vi "Configure Volume.vi"(7 "Save":bool, 8 "error in (no error)":errorcluster, 9 "NumReps":i32, 10 "Scan Settings":T1, 11 "AODAcq in":refnum<class "AODAcq.lvclass">) -> (0 "error out":errorcluster, 3 "AODAcq out":refnum<class "AODAcq.lvclass">)   [LabVIEW 2011, in "AODAcq.lvclass"]
uses:
  AODAcq.lvclass
  <vilib>/rvi/interface/nirviReadWriteControl/nirviReadWriteControl.xnode
  <instrlib>/niHWS/nihws.llb/niHWS Write Analog I32.vi
  FPGA_Control/AODRef.ctl
  FPGA Bitfiles/Acquisition_FPGATarget_AODControl(FPGA)_A1C755F6.lvbitx
  FPGA_Control/AOD Control (FPGA).vi
  <vilib>/rvi/errors/niLvFpgaMergeErrorWithErrorCode.vi
  <vilib>/rvi/errors/niLvFpgaAdjustHostInterfaceError.vi
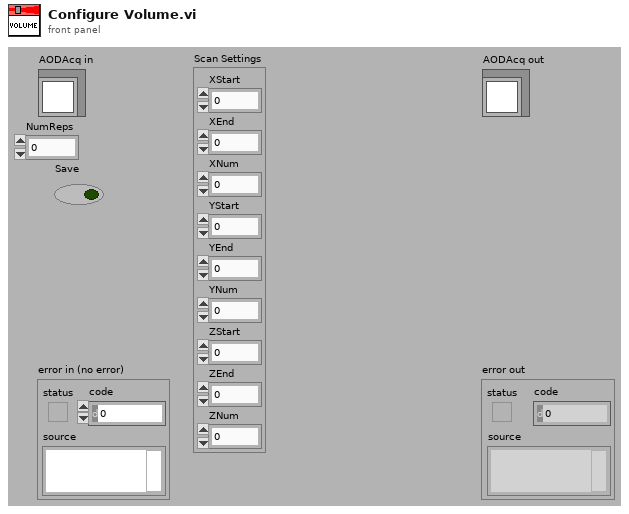
[diagram p1: front panel]
types:
  T1 = cluster{"XStart":i32, "XEnd":i32, "XNum":i32, "YStart":i32, "YEnd":i32, "YNum":i32, "ZStart":i32, "ZEnd":i32, "ZNum":i32}
  T2 = typedef "AODRef.ctl" = refnum<k20>
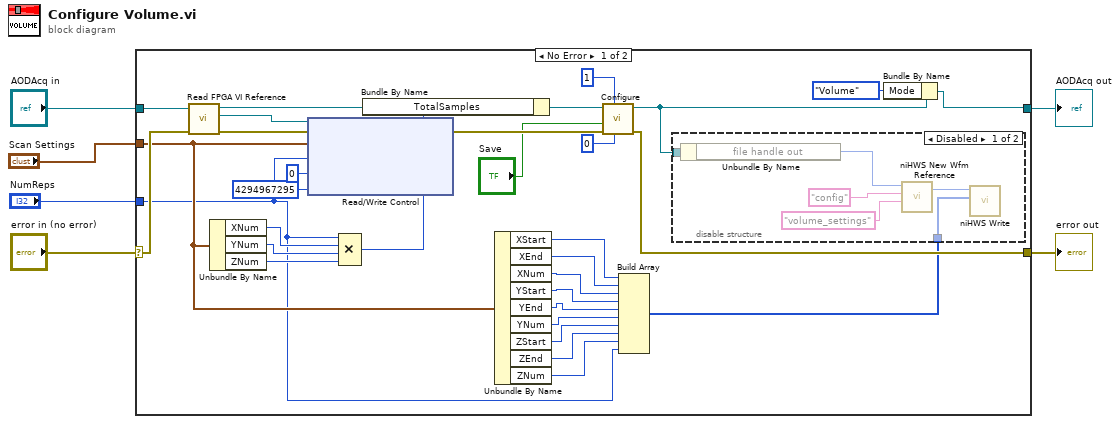
[diagram p0: block diagram]
diagram:
  n1 = case shown="No Error" "error in (no error)" {
    selector: "error in (no error)" -> [w33 w46]
    tunnel: [w32 w46] -> w5
    tunnel: [w11 w45] -> w3
    tunnel: "AODAcq in" -> [w38 w45]
    tunnel: "Scan Settings" -> [w17 _]
    tunnel: "NumReps" -> [w14 _]
    frame No Error {
      n2 = call-dynamic "Read FPGA VI Reference.vi"("error in (no error)"=w33, "AODAcq in"=w38) -> ("error out"=w36:errorcluster, "FPGA VI Reference"=w37:T2, "AODAcq out"=w27:refnum<class "AODAcq.lvclass">)  [unwired: 7 in]
      n3 = Unbundle By Name(w17) -> ("XNum"=w29:i32, "YNum"=w30:i32, "ZNum"=w31:i32)
      n4 = xnode "Read/Write Control"("FPGA VI Reference In"=w37, "error in"=w36, "Scan.VolumeSettings"=w17, "Scan.NumReps"=w14, "Scan.NumMotionPoints"=u32 0, "Scan.Motion Increment"=u32 4294967295) -> ("error out"=w34:errorcluster)  [unwired: 1 out]
      n5 = Compound Arithmetic op=MULTIPLY(w14, w29, w30, w31) -> (w28:i32)
      n6 = Bundle By Name(cluster=w27, "TotalSamples"=w28) -> (w26:refnum<class "AODAcq.lvclass">)
      n7 = Unbundle By Name(w17) -> ("XStart"=w16:i32, "XEnd"=w18:i32, "XNum"=w19:i32, "YStart"=w20:i32, "YEnd"=w21:i32, "YNum"=w22:i32, "ZStart"=w23:i32, "ZEnd"=w24:i32, "ZNum"=w25:i32)
      n8 = call-dynamic "Configure.vi"("GridSize"=u32 0, "Mode"=u32 1, "error in (no error)"=w34, "Save"="Save", "AODAcq in"=w26) -> ("error out"=w32:errorcluster, "AODAcq out"=w13:refnum<class "AODAcq.lvclass">)  [unwired: 5 in]
      n9 = Build Array(w16, w18, w19, w20, w21, w22, w23, w24, w25, w14) -> (w15:i32[])
      n10 = disable-structure shown="Disabled" {
        disable-tunnel: w15 -> [w40 _]
        disable-tunnel: w13 -> [w39 _]
        frame Disabled {
          n11 = Unbundle By Name(w39) -> ("file handle out"=w42:i32)
          n12 = call <instrlib>:"niHWS New Wfm Reference.vi"("waveform name (empty)"="volume_settings", "group name (empty)"="config", "file handle in"=w42) -> ("waveform reference"=w41:u32)  [unwired: 6 in, 2 out]
          n13 = call-poly <instrlib>:"niHWS Write.vi"("data"=w40, "waveform reference in"=w41) -> ()  [unwired: 8 in, 2 out]
        }
        frame Enabled {
        }
      }
      n14 = Bundle By Name(cluster=w13, "Mode"=enum16{"Idle", "Points", "Volume"}."Volume") -> (w11:refnum<class "AODAcq.lvclass">)
    }
    frame Error {
    }
  }
  "error out" <- w5
  "AODAcq out" <- w3
